vi "Query Texture.vi"(11 "Texture Pointer":u32 format="%.0x") -> (0 "Access Pointer":u32 format="%.0x", 1 "Format":u32, 2 "Height":i32, 3 "Width":i32)   [LabVIEW 2015, in "LibSDL2.lvlib"]
uses:
  LibSDL2.lvlib
  DLL/SDL2.dll
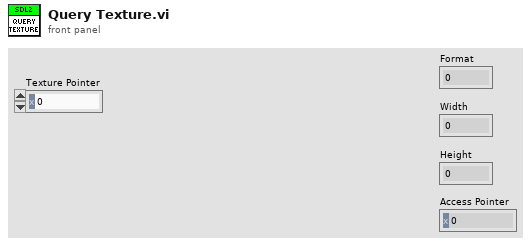
[diagram p1: front panel]
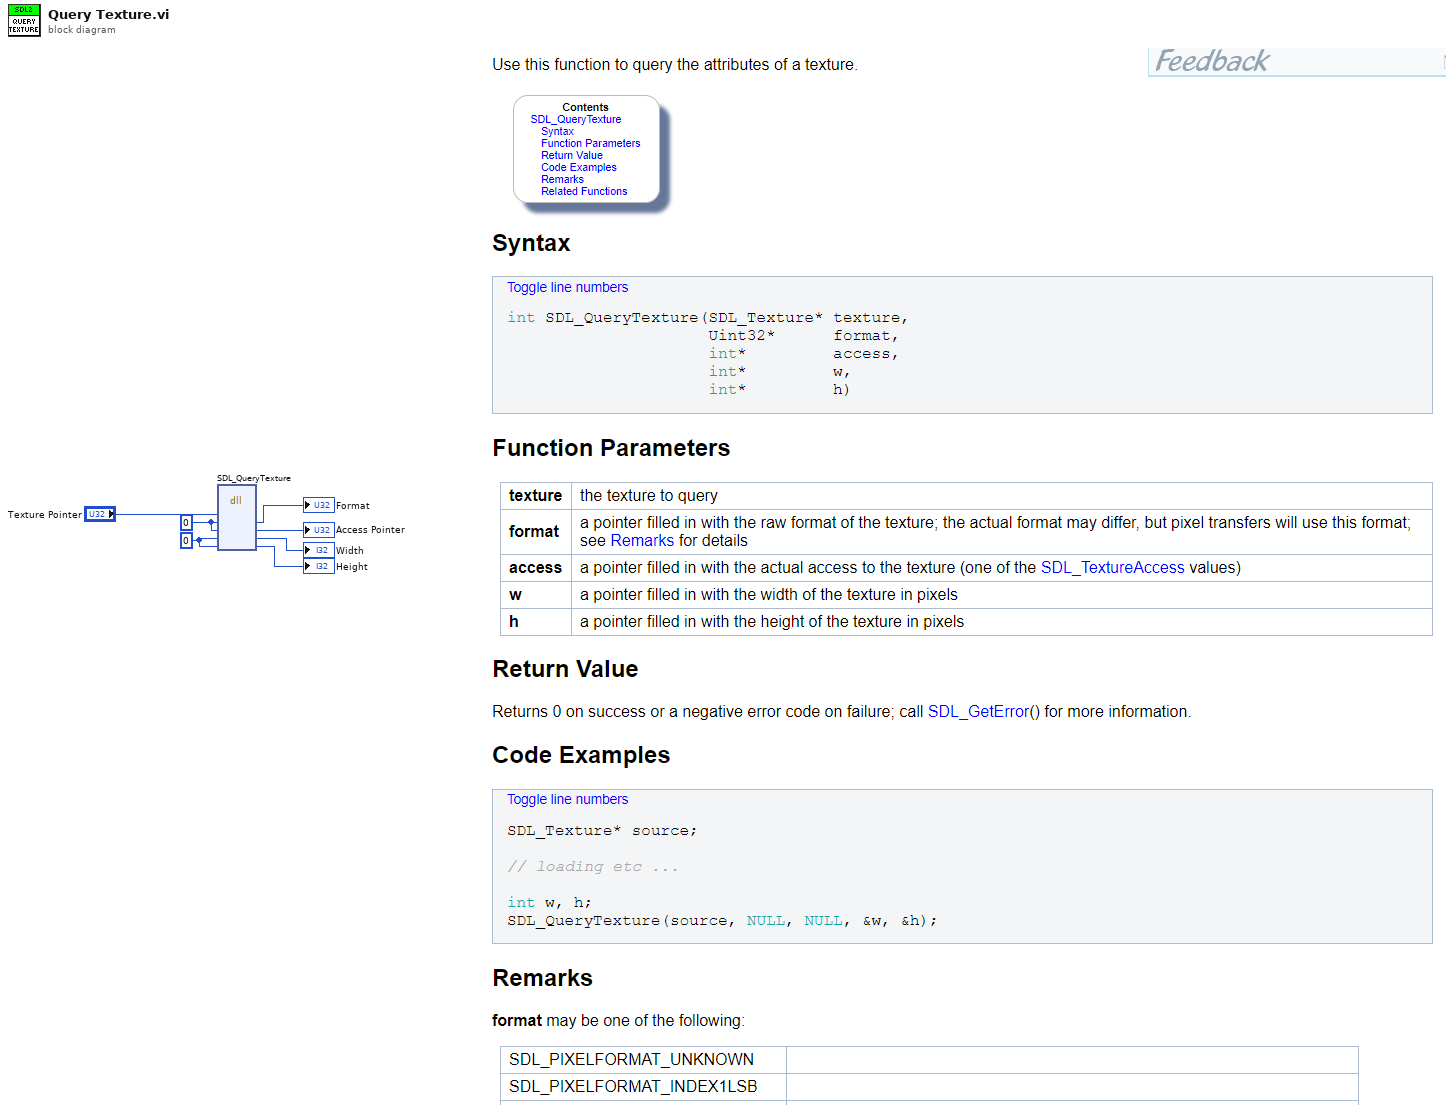
[diagram p0: block diagram]
diagram:
  w6 = 0 ("width")
  w4 = u32 0 ("format")
  n1 = dll-call lib="C:/dev/PGS/LabSDL2/Source/Libraries/LibSDL2 Wrapper/DLL/SDL2.dll" fn="SDL_QueryTexture"("texture"="Texture Pointer", "format"=w4, "access"=w4, "width"=w6, "height"=w6) -> ("format"=→"Format":u32, "access"=→"Access Pointer":u32, "width"=→"Width":i32, "height"=→"Height":i32)  [unwired: 5 in, 2 out]
